vi "XIPIN_802.16e_CTC_Decoder_4_0.vi"   [LabVIEW 2017]
doc: "The 802.16e CTC Decoder LogiCORE is a drop-in module for Virtex-4(TM), Virtex-5(TM), Virtex-6(TM), Spartan-3(TM), Spartan-3E(TM), Spartan-3A DSP(TM) and Spartan-6(TM) families of FPGA. It performs iterative soft decoding of channel data that has been encoded as described in Section 8.4.9.2.3 of the IEEE Std 802.16e-2005 specification and the corrigendum IEEE P802.16Rev2/D0b (June 2007). The core is fully synchronous, using a single clock, and integrates seamlessly with the Xilinx design flow.\n------------------------------------\n<b>Need License</b> : Yes"
uses:
  <vilib>/rvi/XilinxIP/XIPIN_XNode/niFpgaXIPIN.xnode
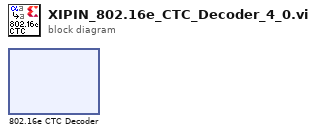
[diagram p0: block diagram]
diagram:
  n1 = xnode ("802.16e CTC Decoder")() -> ()
